vi "FlatToRichexternal_driver_wrapper_ConfigureMeasurementDigitsRequest.vi"(5 "OutputClusterType":T1, 11 "InputCluster":T2) -> (3 "OutputCluster":T1)   [LabVIEW 2020, in "Instrument Interaction Client.lvlib"]
uses:
  Instrument Interaction Client.lvlib
  external_driver_wrapper_ConfigureMeasurementDigitsRequest_Flat.ctl
  external_driver_wrapper_ConfigureMeasurementDigitsRequest.ctl
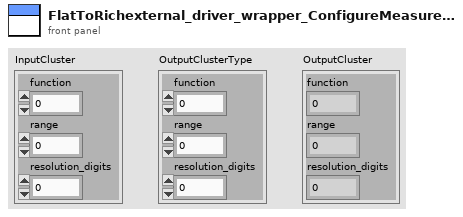
[diagram p1: front panel]
types:
  T1 = typedef "Instrument Interaction Client.lvlib/external_driver_wrapper_ConfigureMeasurementDigitsRequest.ctl" = cluster{"function":i32, "range":dbl, "resolution_digits":dbl}
  T2 = typedef "Instrument Interaction Client.lvlib/external_driver_wrapper_ConfigureMeasurementDigitsRequest_Flat.ctl" = cluster{"function":i32, "range":dbl, "resolution_digits":dbl}
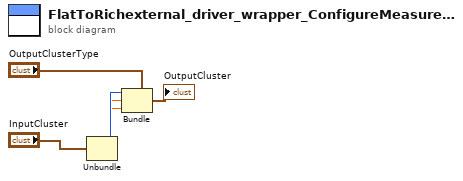
[diagram p0: block diagram]
diagram:
  n1 = Unbundle "Unbundle"("InputCluster") -> ("function"=w3:i32, "range"=w2:dbl, "resolution_digits"=w1:dbl)
  n2 = Bundle "Bundle"(cluster="OutputClusterType", "function"=w3, "range"=w2, "resolution_digits"=w1) -> (→"OutputCluster":T1)
